vi "Disconnect.vi"(8 "error in":errorcluster, 11 "Acopian in":refnum<class "Acopian.lvclass">) -> (0 "error out":errorcluster, 3 "Acopian out":refnum<class "Acopian.lvclass">)   [LabVIEW 2019, in "Acopian.lvlib" / "Acopian.lvclass"]
uses:
  Library/Acopian.lvclass
  Library/Acopian.lvclass/Acopian.ctl
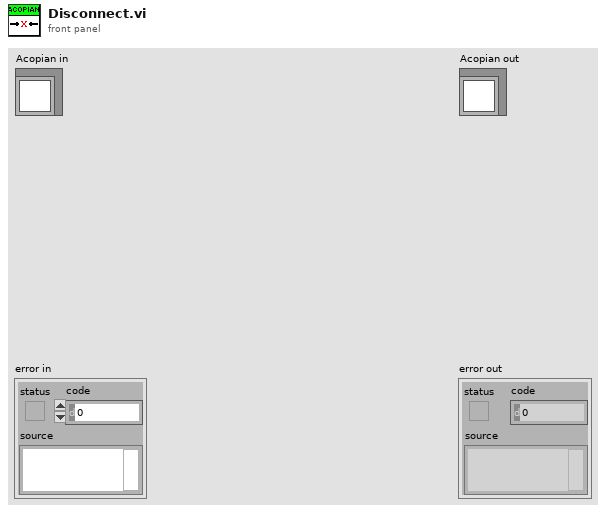
[diagram p1: front panel]
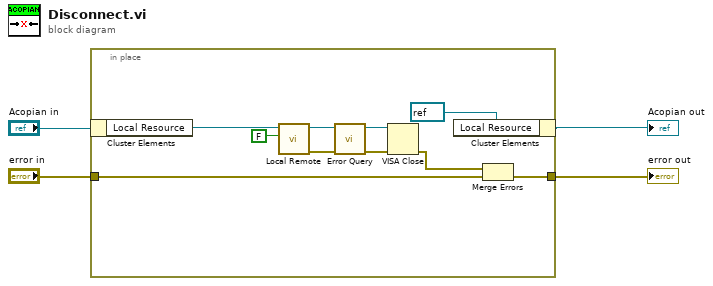
[diagram p0: block diagram]
diagram:
  n1 = in-place {
    in-place-border: "error in" -> [w6]
    in-place-border: [w5] -> w1
    n2 = in-place-cluster #1("Acopian in") -> ("Local Resource"=w9:refnum<visa-resource-name>)
    n3 = call "Local Remote.vi"("Remote (T: Remote)"=FALSE, "VISA resource name"=w9) -> ("error out"=w13:errorcluster, "VISA resource out"=w12:refnum<visa-resource-name>)  [unwired: 8 in]
    n4 = call "Error Query.vi"("error in"=w13, "VISA resource in"=w12) -> ("error out"=w11:errorcluster, "VISA resource out"=w10:refnum<visa-resource-name>)  [unwired: 6 in, 2 out]
    n5 = VISA Close(VISA resource name=w10, error in (no error)=w11) -> (error out=w7:errorcluster)
    n6 = in-place-cluster #1("Local Resource"=refnum<visa-resource-name> refnum) -> (→"Acopian out":refnum<class "Acopian.lvclass">)
    n7 = Merge Errors(w7, w6) -> (w5:errorcluster)
  }
  "error out" <- w1
